vi "ROI grp-ROI groups window refresh signal.vi"(8 "error in (no error)":errorcluster) -> (0 "error out":errorcluster)   [LabVIEW 2020]
uses:
  Globals/gl_ROI grp window globals.vi
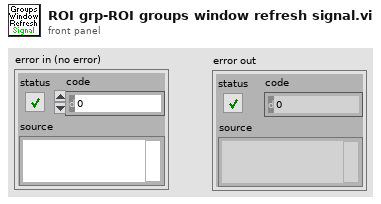
[diagram p1: front panel]
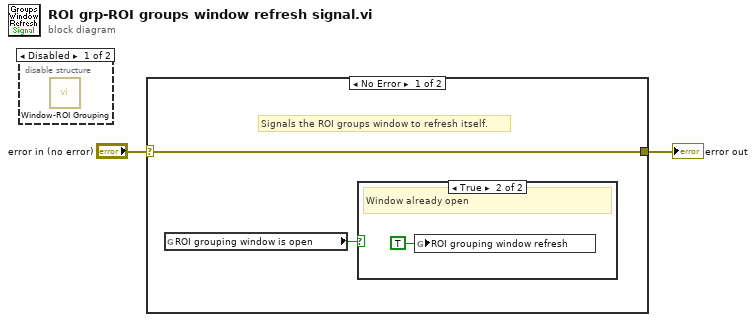
[diagram p0: block diagram]
diagram:
  n1 = disable-structure shown="Disabled" {
    frame Disabled {
      n2 = call "Window-ROI Grouping.vi"() -> ()  [unwired: 12 in]
    }
    frame Enabled {
    }
  }
  n3 = case shown="No Error" "error in (no error)" {
    selector: "error in (no error)" -> [w3 w6]
    tunnel: [w3 w6] -> w1
    frame No Error {
      # "Signals the ROI groups window to refresh itself."
      n4 = global read "gl_ROI grp window globals.vi" "ROI grouping window is open"() -> (w4:bool)
      n5 = case shown="True" w4 {
        frame False {
          # "Window is not open"
        }
        frame True {
          # "Window already open"
          n6 = global write "gl_ROI grp window globals.vi" "ROI grouping window refresh"(TRUE ("Groups vis window refresh")) -> ()
        }
      }
    }
    frame Error {
    }
  }
  "error out" <- w1
